vi "2D experiment wii.vi"() -> ()   [LabVIEW 2011]
uses:
  <vilib>/Platform/TimedLoop/XDataNode/timing_clust.ctl
  <vilib>/Platform/TimedLoop/XDataNode/nitl_modes.ctl
  <vilib>/Platform/TimedLoop/XDataNode/wakeup.ctl
  3D_Experiment/libs/experiments 2/Action Engines/AE Access VIs/AE - Bluetooth Initialise.vi
  3D_Experiment/libs/experiments 2/Action Engines/AE Access VIs/AE - Bluetooth Connect All.vi
  <vilib>/Utility/cursorutil.llb/Set Cursor (Cursor ID).vi
  <vilib>/Utility/inputDevices.llb/closeMouse.vi
  <vilib>/Utility/inputDevices.llb/mouseAcquire.vi
  <vilib>/Utility/file.llb/Write To Spreadsheet File (DBL).vi
  <vilib>/Utility/file.llb/Write To Spreadsheet File (I64).vi
  <vilib>/Platform/TimedLoop/XDataNode/XDataNode.xnode
  User32.dll
  <vilib>/Platform/TimedLoop/XDataNode/XDNodeRunTimeDep.lvlib
panel:
  out "initial time":u32
  out "XY Graph":cluster{"Y":dbl[], "Y":dbl[]}[](graph)
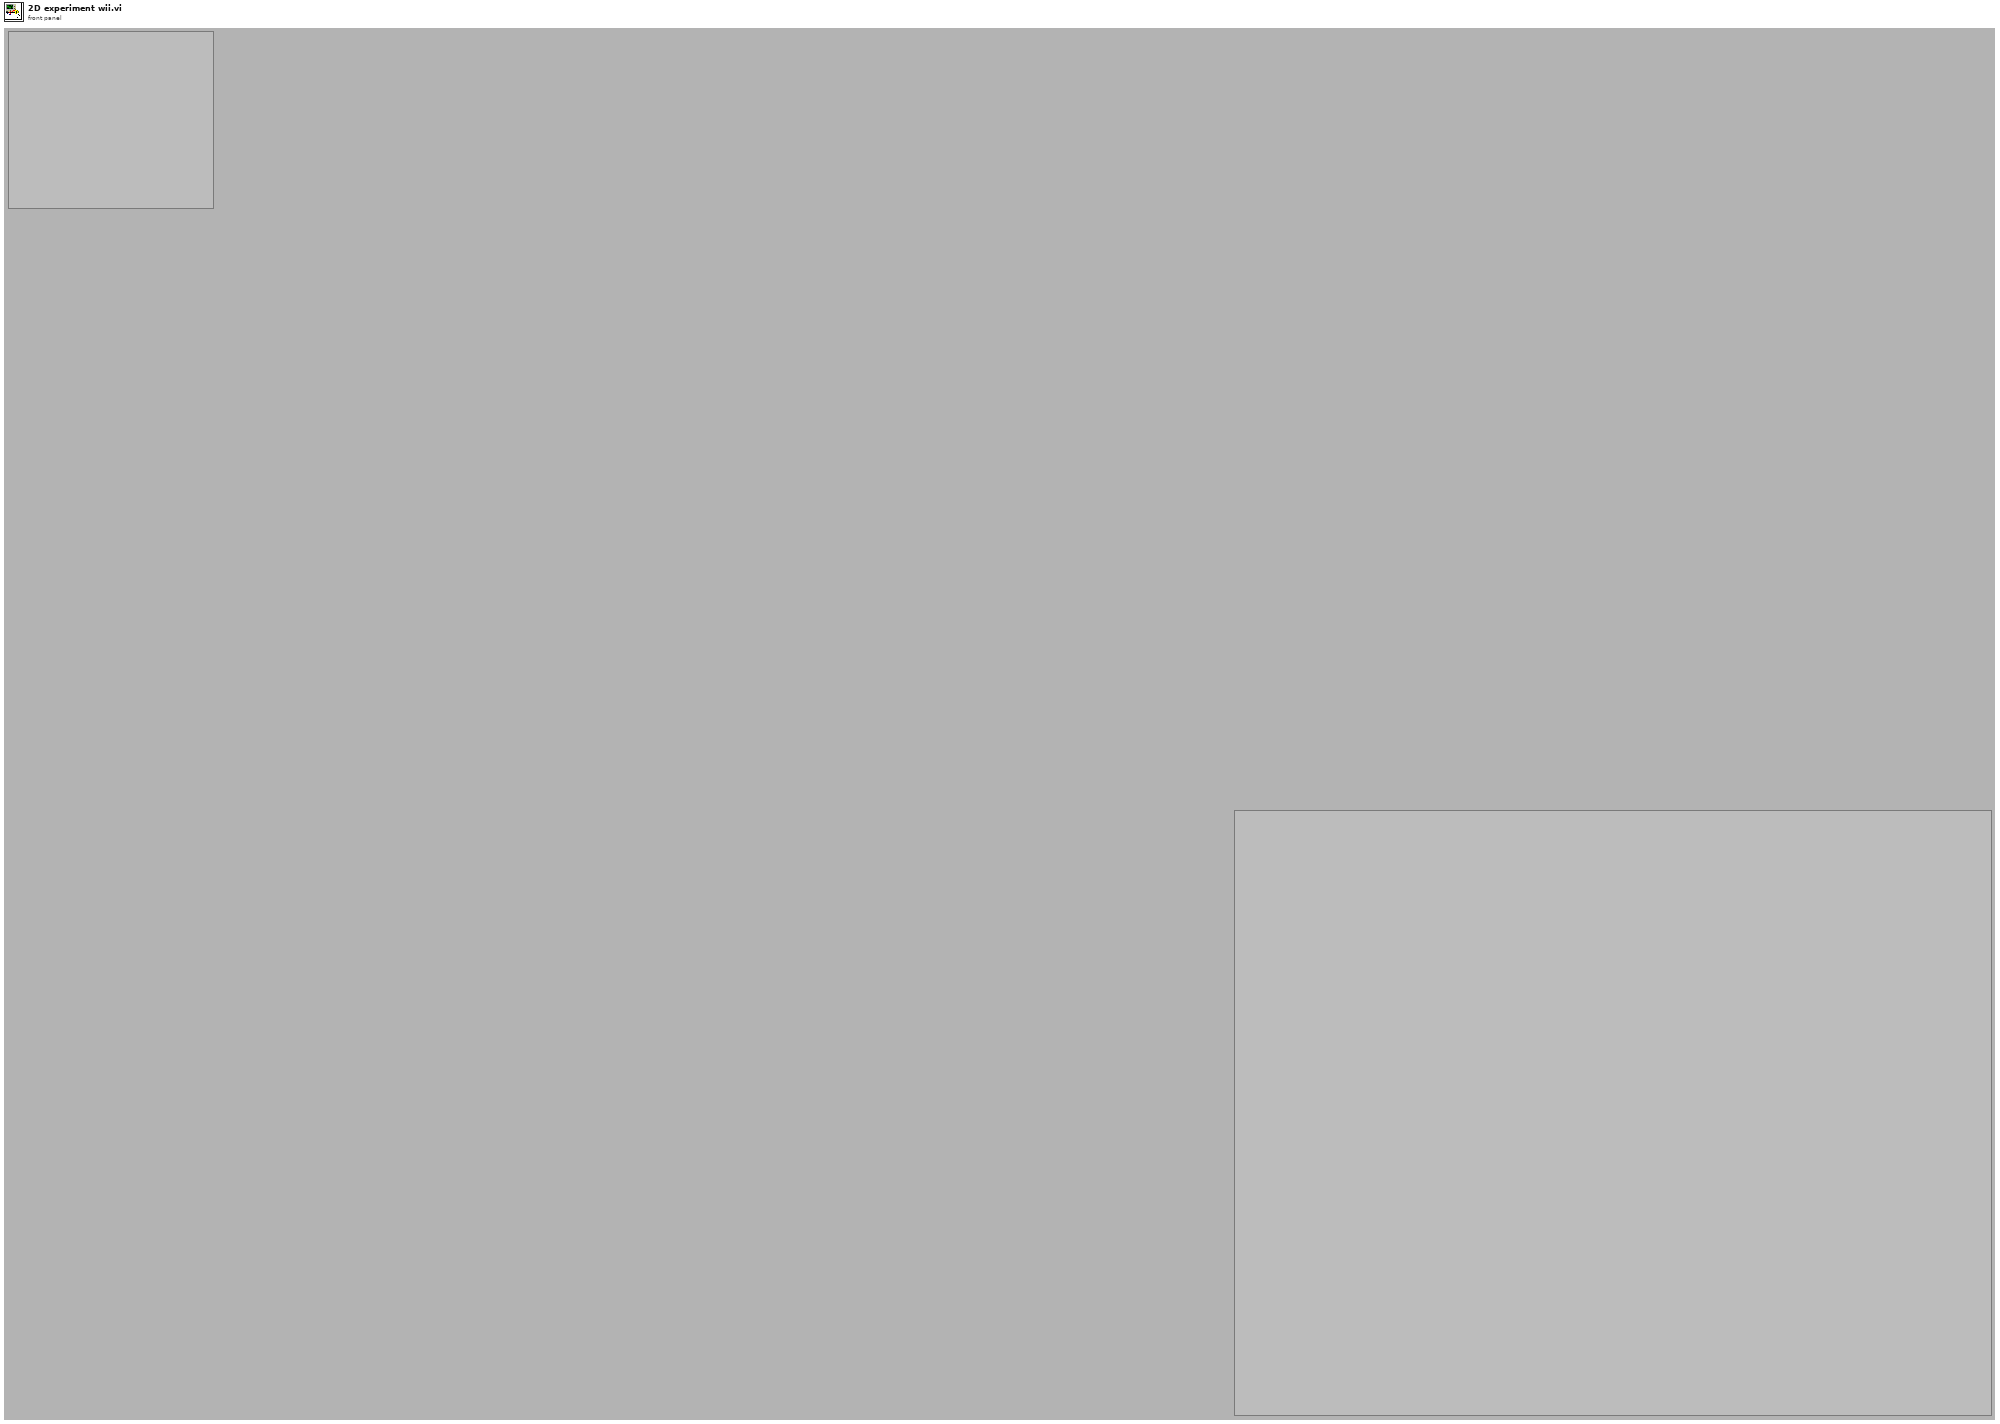
[diagram p1: front panel]
types:
  T1 = enum16{"open", "replace", "create", "open or create", "replace or create", "replace or create with confirmation"}
  T2 = typedef "XDNodeRunTimeDep.lvlib/timing_clust.ctl" = cluster{"Expected End [f-1]":u64, "Actual End [f-1]":u64, "Finished Late? [f-1]":bool, "Expected End [i-1]":u64, "Actual End [i-1]":u64, "Finished Late? [i-1]":bool, "Expected Start [i]":u64, "Actual Start [i]":u64, "Expected Start [f]":u64, "Actual Start [f]":u64, "Source Name":string, "Structure Name":string, "Period":i64, "Deadline":i64, "Offset":i64, "Start":i64, "Priority":i32, "Timeout":i32, "Mode":T3, "Wakeup Reason":T4, "Error":errorcluster, "Source Type":string, "Secondary Source Type":string, "Global End Time":u64, "Global Start Time":u64, "Frame Duration":u64, "Iteration Duration":u64, "Assigned CPU":i32, "I/O Scan Engine Mode":u32}
  T3 = typedef "XDNodeRunTimeDep.lvlib/nitl_modes.ctl" = enum32{"No Change", "Process missed periods, maintain original phase", "Discard missed periods, maintain original phase", "Process missed periods, ignore original phase", "Discard missed periods, ignore original phase"}
  T4 = typedef "XDNodeRunTimeDep.lvlib/wakeup.ctl" = enum32{"Normal", "Aborted", "Asynchronous wakeup", "Timing source error", "Timed loop error", "Timeout"}
  T5 = typedef "LVAllMonitorsDisplayTypeDef.ctl" = cluster{"Bounds":cluster{"Left":i16, "Top":i16, "Right":i16, "Bottom":i16}, "Depth":i16}[]
  T6 = cluster{"Bounds":cluster{"Left":i16, "Top":i16, "Right":i16, "Bottom":i16}, "Depth":i16}
  T7 = cluster{"Left":i16, "Top":i16, "Right":i16, "Bottom":i16}
  T8 = cluster{"Horizontal":i32, "Vertical":i32, "Scrolling":i32}
  T9 = cluster{"button 1":bool, "button 2":bool, "button 3":bool, "button 4":bool}
  T10 = cluster{"Radius":dbl, "x0":dbl, "y0":dbl, "D":dbl, bool}
  T11 = typedef "LVPoint32TypeDef.ctl" = cluster{"Horizontal":i32, "Vertical":i32}
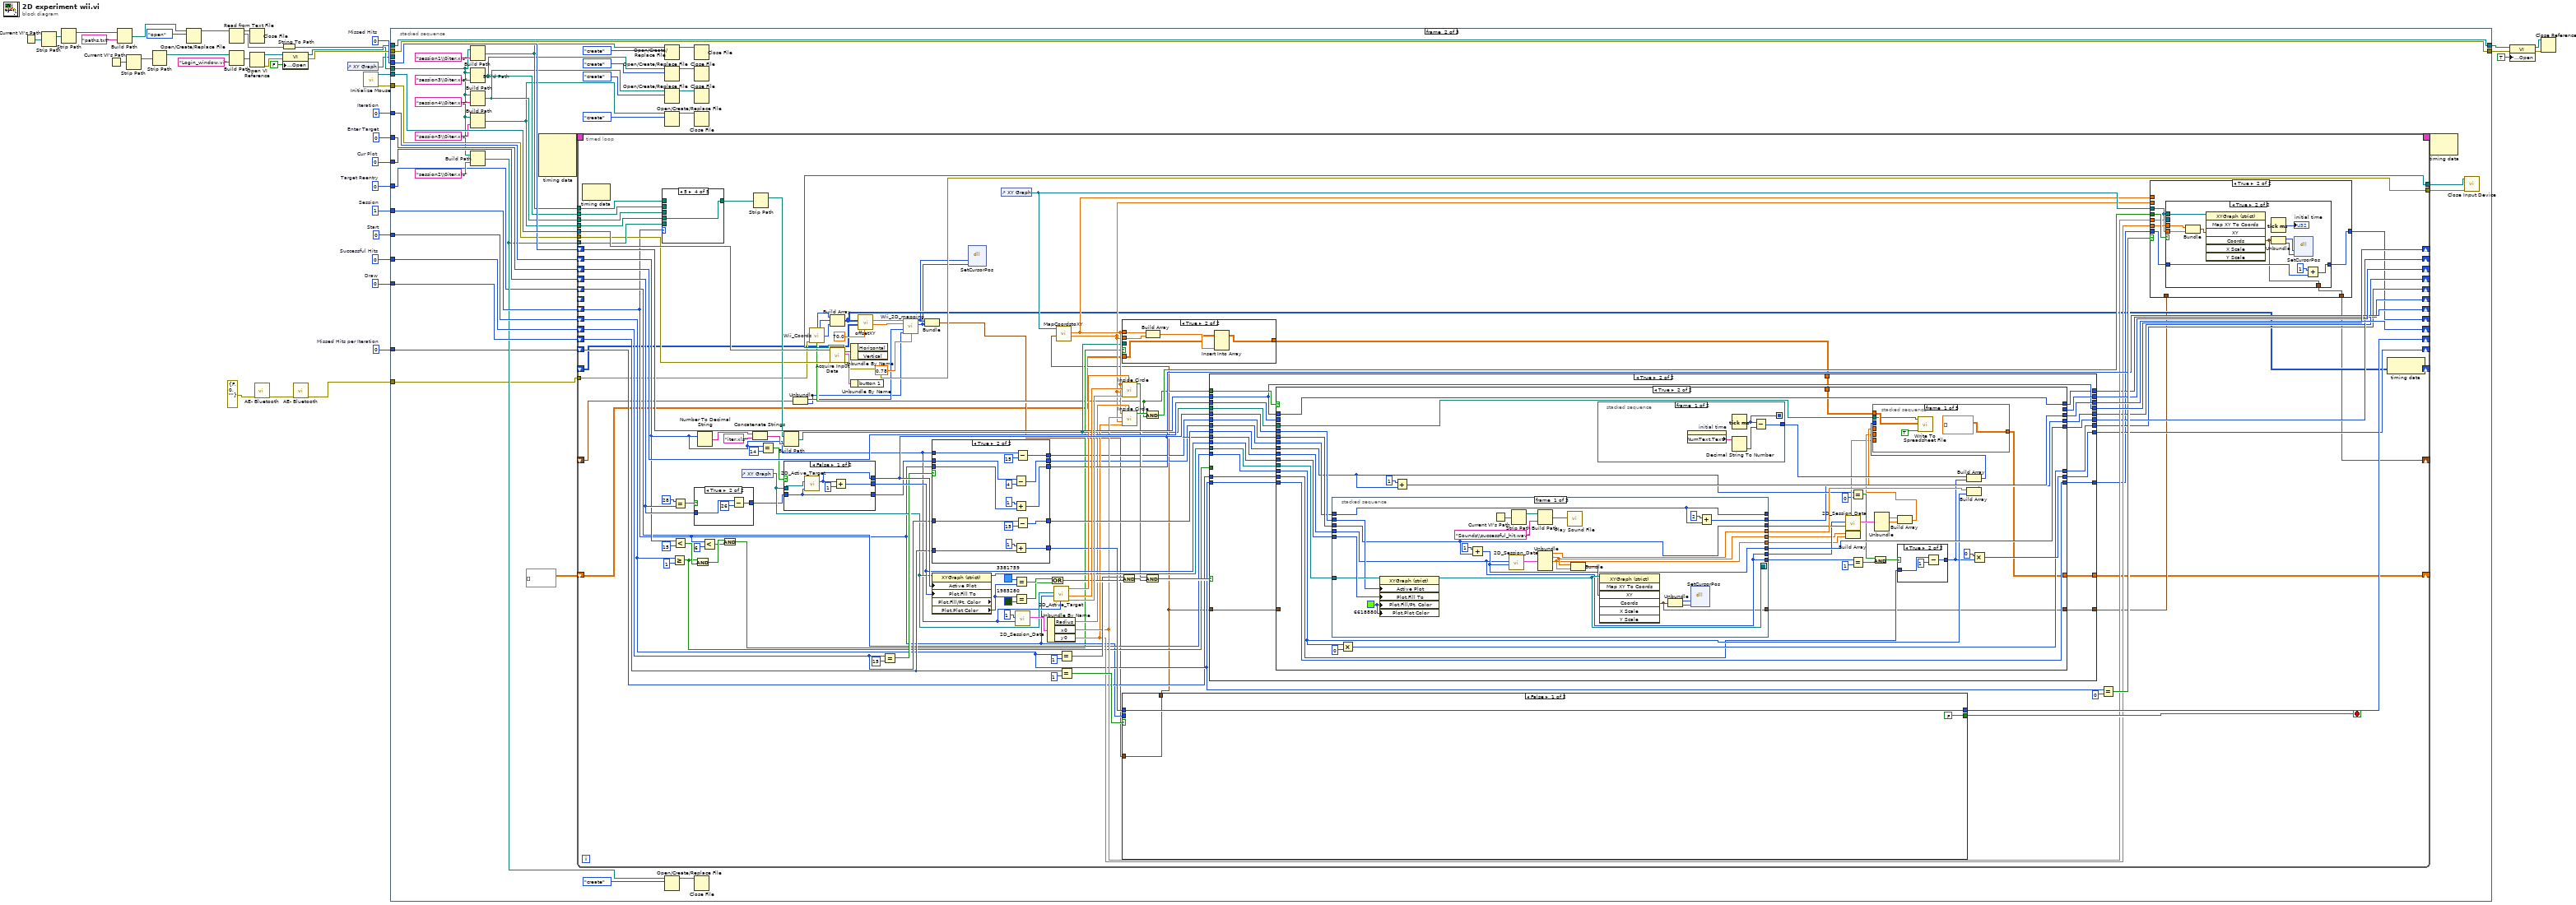
[diagram p0: block diagram]
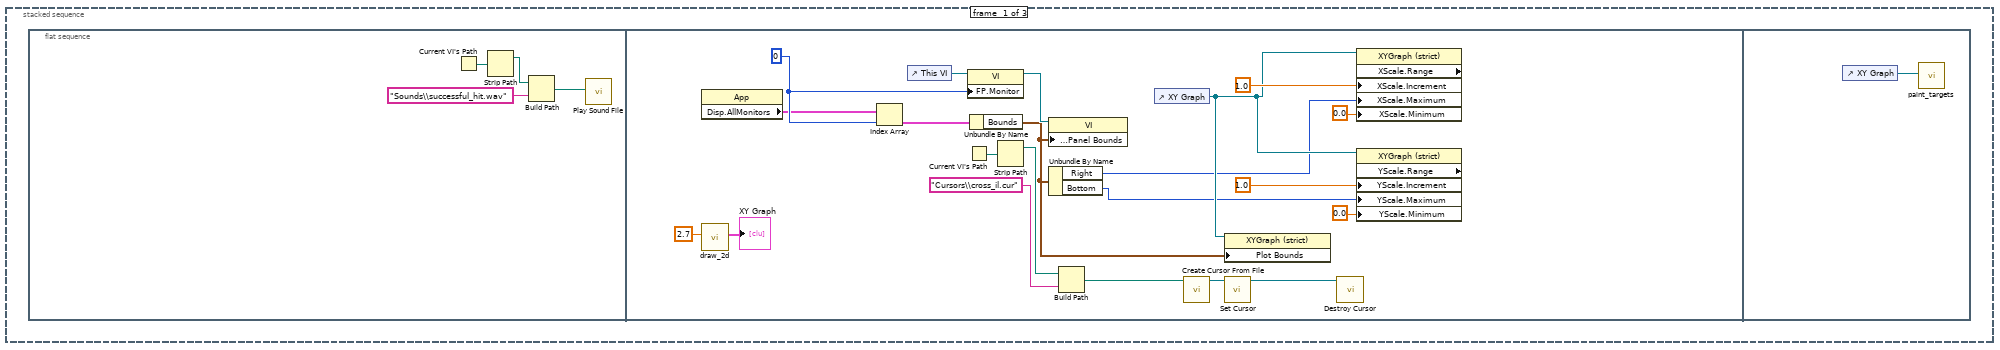
[diagram p2: hidden frame]
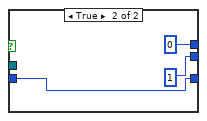
[diagram p8: hidden frame]
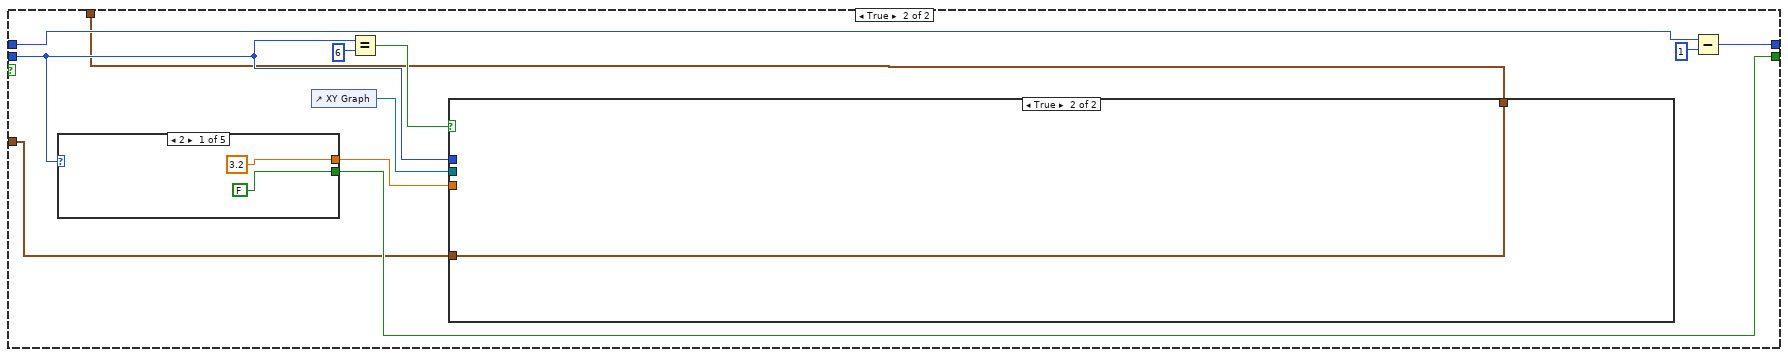
[diagram p10: hidden frame]
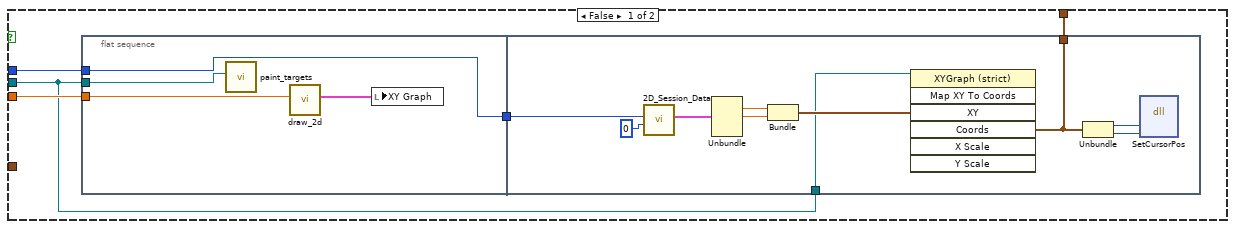
[diagram p11: hidden frame]
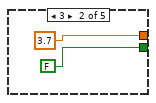
[diagram p12: hidden frame]
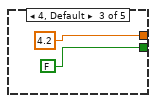
[diagram p13: hidden frame]
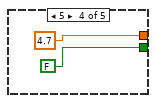
[diagram p14: hidden frame]
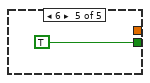
[diagram p15: hidden frame]
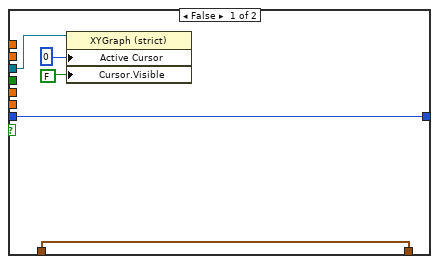
[diagram p16: hidden frame]
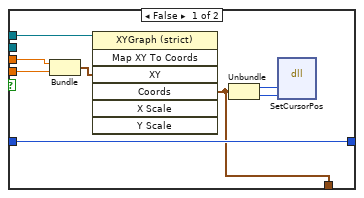
[diagram p17: hidden frame]
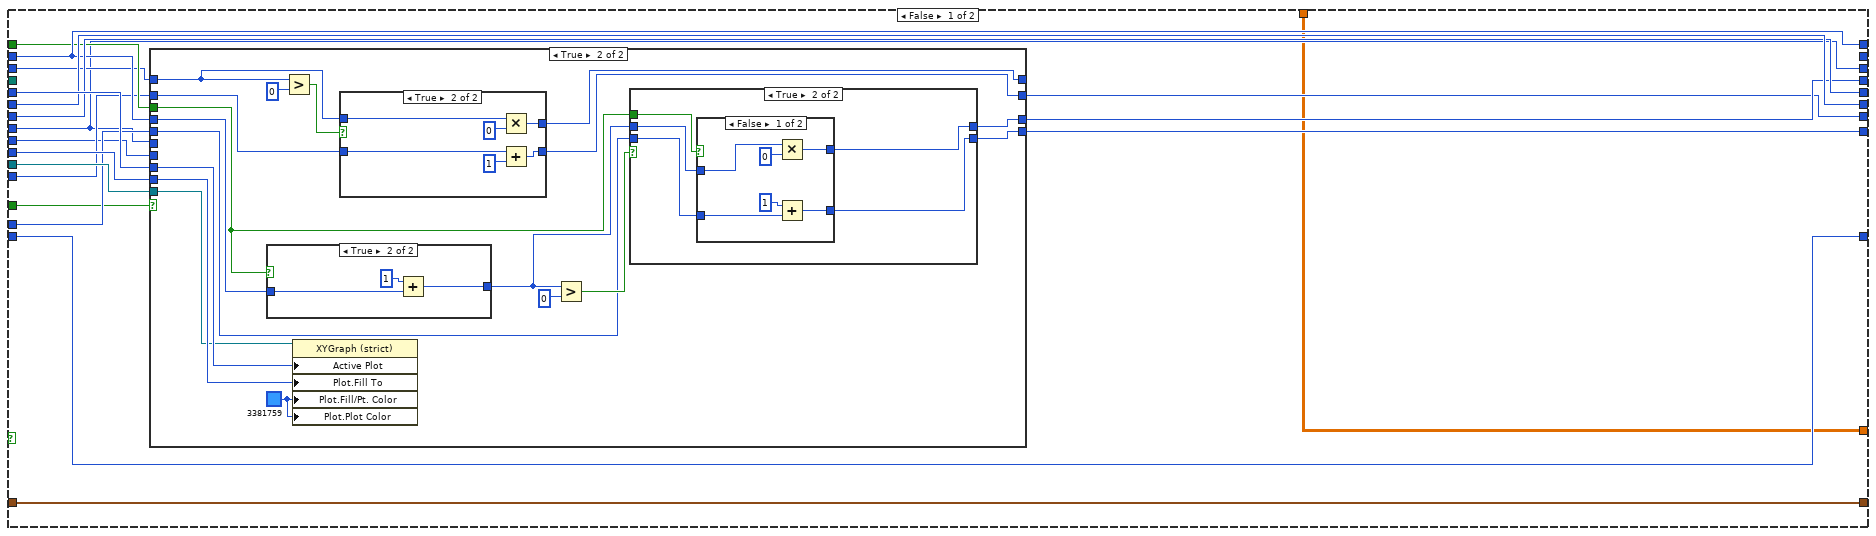
[diagram p19: hidden frame]
diagram:
  w4 = 0  # Target Reentry
  w5 = 0  # Missed Hits per Iteration
  w33 = 0  # Iteration
  w34 = 0  # Cur Plot
  w36 = 0  # Start
  w37 = 0  # Draw
  w38 = 1  # Session
  w39 = 0  # Successful Hits
  w40 = 0  # Missed Hits
  w41 = 0  # Enter Target
  n1 = Current VI's Path() -> (path=w14:path)
  n2 = Strip Path(path=w14) -> (stripped path=w9:path)  [unwired: 1 out]
  n3 = Strip Path(path=w9) -> (stripped path=w8:path)  [unwired: 1 out]
  n4 = Current VI's Path() -> (path=w29:path)
  n5 = Build Path(base path=w8, name or relative path="paths.txt") -> (appended path=w13:path)
  n6 = Strip Path(path=w29) -> (stripped path=w24:path)  [unwired: 1 out]
  n7 = Strip Path(path=w24) -> (stripped path=w23:path)  [unwired: 1 out]
  n8 = Open/Create/Replace File(file path (use dialog)=w13, operation (0:open)=T1."open") -> (refnum out=w16:refnum<file>)  [unwired: 4 in, 2 out]
  n9 = Read from Text File(file (use dialog)=w16) -> (refnum out=w17:refnum<file>, text=w15:string)  [unwired: 3 in, 2 out]
  n10 = Build Path(base path=w23, name or relative path="Login_window.vi") -> (appended path=w27:path)
  n11 = Close File(refnum=w17) -> ()  [unwired: 1 in, 2 out]
  n12 = Open VI Reference(vi path=w27) -> (vi reference=w32:refnum<vi>, error out=w31:errorcluster)  [unwired: 5 in]
  n13 = call-poly "AE- Bluetooth.vi"("error in (no error)"=errorcluster {"status"=FALSE, "code"=0, "source"=""}) -> ("error out"=w3:errorcluster)  [unwired: 10 in]
  n14 = String To Path(string=w15) -> (path=w10:path)
  n15 = property class="VI"(reference=w32, error in=w31, "Front Panel Window:Open"=FALSE) -> (reference out=w26:refnum<vi>, error out=w25:errorcluster)
  n16 = call-poly "AE- Bluetooth.vi"("error in (no error)"=w3) -> ("error out"=w2:errorcluster)  [unwired: 9 in, 1 out]
  n17 = control-ref of="XY Graph"() -> (w7:refnum<vi>)
  n18 = call <vilib>:"Initialize Mouse.vi"() -> ("error out"=w6:errorcluster, "device ID"=w35:refnum<k1>)  [unwired: 10 in]
  n19 = stacked-sequence {
    tunnel: w35 -> [_ w108 _]
    tunnel: w39 -> [_ w107 _]
    tunnel: w40 -> [_ w106 _]
    tunnel: w38 -> [_ w102 _]
    tunnel: w36 -> [_ w105 _]
    tunnel: w37 -> [_ w104 _]
    tunnel: w41 -> [_ w103 _]
    tunnel: w34 -> [_ w101 _]
    tunnel: w33 -> [_ w100 _]
    tunnel: w26 -> [_ w97 _]
    tunnel: w25 -> [_ w96 _]
    tunnel: [_ w97 _] -> w19
    tunnel: [_ w96 _] -> w18
    tunnel: w10 -> [_ w76 _]
    tunnel: w7 -> [_ _ w568]
    tunnel: w6 -> [_ w82 _]
    tunnel: w5 -> [_ w80 _]
    tunnel: w4 -> [_ w79 _]
    tunnel: w2 -> [_ w69 _]
    frame #0 {
      n20 = flat-sequence {
        frame #0 {
          n21 = Current VI's Path() -> (path=w43:path)
          n22 = Strip Path(path=w43) -> (stripped path=w44:path)  [unwired: 1 out]
          n23 = Build Path(base path=w44, name or relative path="Sounds\\successful_hit.wav") -> (appended path=w42:path)
          n24 = call <vilib>:"Play Sound File.vi"("path"=w42) -> ()  [unwired: 9 in, 2 out]
        }
        frame #1 {
          w62 = u16 0 ("Front Panel Window:Monitor")
          n25 = property class="App"() -> ("Disp.AllMonitors"=w61:T5)  [unwired: 2 in, 2 out]
          n26 = call "draw_2d.vi"("ID"=2.7) -> ("appended array"=→"XY Graph":cluster{dbl[], dbl[]}[])  [unwired: 10 in]
          n27 = Index Array(array=w61, index=w62) -> (element=w63:T6)
          n28 = control-ref of="This VI"() -> (w64:refnum<vi>)
          n29 = Current VI's Path() -> (path=w53:path)
          n30 = property class="VI"(reference=w64, "FP.Monitor"=w62) -> (reference out=w60:refnum<vi>)  [unwired: 1 in, 1 out]
          n31 = Unbundle By Name(w63) -> ("Bounds"=w59:T7)
          n32 = Strip Path(path=w53) -> (stripped path=w52:path)  [unwired: 1 out]
          n33 = property class="VI"(reference=w60, "Front Panel Window:Panel Bounds"=w59) -> ()  [unwired: 1 in, 2 out]
          n34 = Unbundle By Name(w59) -> ("Right"=w47:i16, "Bottom"=w46:i16)
          n35 = Build Path(base path=w52, name or relative path="Cursors\\cross_il.cur") -> (appended path=w50:path)
          n36 = control-ref of="XY Graph"() -> (w54:refnum<vi>)
          n37 = call <vilib>:"Create Cursor From File.vi"("cursor file"=w50) -> ("cursor ID"=w49:refnum<k1>)  [unwired: 9 in, 1 out]
          n38 = property on="Property Node" class="XYGraph (strict)"(reference=w54, "Plot Bounds"=w59) -> ()  [unwired: 1 in, 2 out]
          n39 = call-poly <vilib>:"Set Cursor.vi"("cursor ID"=w49) -> ("previous cursor ID"=w48:refnum<k1>)  [unwired: 9 in, 1 out]
          n40 = call <vilib>:"Destroy Cursor.vi"("cursor ID"=w48) -> ()  [unwired: 9 in, 1 out]
          n41 = property on="Property Node" class="XYGraph (strict)" props=["XScale", "Range", "XScale", "Increment", "XScale", "Maximum", "XScale", "Minimum"](reference=w54, "XScale.Increment"=1.0 ("X Scale.Range:Increment"), "XScale.Maximum"=w47, "XScale.Minimum"=0.0 ("X Scale.Range:Minimum")) -> ()  [unwired: 1 in, 3 out]
          n42 = property on="Property Node" class="XYGraph (strict)" props=["YScale", "Range", "YScale", "Increment", "YScale", "Maximum", "YScale", "Minimum"](reference=w54, "YScale.Increment"=1.0 ("Y Scale.Range:Increment"), "YScale.Maximum"=w46, "YScale.Minimum"=0.0 ("Y Scale.Range:Minimum")) -> ()  [unwired: 1 in, 3 out]
        }
        frame #2 {
          n43 = control-ref of="XY Graph"() -> (w67:refnum<vi>)
          n44 = call "paint_targets.vi"("XYGraph Refnum"=w67) -> ()  [unwired: 11 in]
        }
      }
    }
    frame #1 {
      n45 = Build Path(base path=w76, name or relative path="session1\\0iter.xls") -> (appended path=w90:path)
      n46 = Build Path(base path=w76, name or relative path="session3\\0iter.xls") -> (appended path=w84:path)
      n47 = Build Path(base path=w76, name or relative path="session4\\0iter.xls") -> (appended path=w73:path)
      n48 = Build Path(base path=w76, name or relative path="session5\\0iter.xls") -> (appended path=w70:path)
      n49 = Build Path(base path=w76, name or relative path="session2\\0iter.xls") -> (appended path=w87:path)
      n50 = node-c288() -> (w99:T2)  [unwired: 4 in]
      n51 = timed-loop {
        tunnel: w108 -> [w213]
        tunnel: [w212] -> w83
        shift-right: [w211] -> _
        shift-left: w107 -> [w198]
        shift-right: [w209] -> _
        shift-left: w106 -> [w210]
        shift-right: [w190] -> _
        shift-left: w102 -> [w137]
        shift-right: [w139] -> _
        shift-left: w105 -> [w158]
        shift-right: [w195] -> _
        shift-left: w104 -> [w196]
        shift-right: [w191] -> _
        shift-left: w103 -> [w192]
        shift-right: [w175] -> _
        shift-left: w100 -> [w149]
        shift-right: [w174] -> _
        shift-left: w101 -> [w171]
        timing: w99 -> [_]
        timing-out: [_] -> w98
        tunnel: w90 -> [w164]
        tunnel: w87 -> [w163]
        tunnel: w84 -> [w162]
        shift-right: [w151] -> _
        shift-left: _ -> [_]
        tunnel: w82 -> [w147]
        tunnel: [w146] -> w81
        shift-right: [w144] -> _
        shift-left: w80 -> [w145]
        shift-right: [w141] -> _
        shift-left: w79 -> [w143]
        tunnel: w73 -> [w133]
        tunnel: w70 -> [w132]
        tunnel: w69 -> [w123]
        shift-right: [w122] -> _
        shift-left: _ -> [w121]
        shift-right: [w117] -> _
        shift-left: _ -> [w116]
        shift-right: [w109] -> _
        shift-left: dbl[][] [] -> [w111]
        stop <- w184 stop-if-true
        n52 = node-c288() -> ()  [unwired: 1 in, 1 out]
        n53 = case shown="5" w137 {
          tunnel: w164 -> [_ _ _ _ w234]
          tunnel: [w230 w231 w232 w233 w234] -> w157
          tunnel: w163 -> [w230 _ _ _ _]
          tunnel: w162 -> [_ w231 _ _ _]
          tunnel: w133 -> [_ _ w232 _ _]
          tunnel: w132 -> [_ _ _ w233 _]
          frame 2 {
          }
          frame 3 {
          }
          frame 4 {
          }
          frame 5 {
          }
          frame 1, Default {
          }
        }
        n54 = Greater Or Equal?(x=w158, y=1) -> (x >= y?=w142:bool)
        n55 = Equal?(x=28, y=w171) -> (x = y?=w172:bool)
        n56 = Less?(x=w149, y=15) -> (x < y?=w148:bool)
        n57 = case shown="True" w172 {
          tunnel: w171 -> [w245 w248]
          tunnel: [w245 w246] -> w170
          frame False {
          }
          frame True {
            n58 = Subtract(x=w248, y=26) -> (x-y=w246:i32)
          }
        }
        n59 = And(x=w142, y=w148) -> (x .and. y?=w138:bool)
        n60 = Number To Decimal String(number=w149) -> (decimal integer string=w153:string)  [unwired: 1 in]
        n61 = Less?(x=w137, y=6) -> (x < y?=w135:bool)
        n62 = And(x=w138, y=w135) -> (x .and. y?=w134:bool)
        n63 = control-ref of="XY Graph"() -> (w178:refnum<vi>)
        n64 = Concatenate Strings(w153, "iter.xls" ("name or relative path")) -> (w155:string)
        n65 = Strip Path(path=w157) -> (stripped path=w154:path)  [unwired: 1 out]
        n66 = Equal?(x=w149, y=14) -> (x = y?=w168:bool)
        n67 = Build Path(base path=w154, name or relative path=w155) -> (appended path=w152:path)
        n68 = case shown="False" w168 {
          tunnel: [w240 u32 0 ("Active Plot")] -> w218
          tunnel: [w239 u32 1] -> w217
          tunnel: w178 -> [w238 _]
          tunnel: w170 -> [w237 w242]
          tunnel: [w237 w242] -> w167
          frame False {
            n69 = call "2D_Active_Target.vi"("Active Plot"=w237, "XYGraph Refnum"=w238) -> ("Active Plot"=w240:u32)  [unwired: 6 in, 3 out]
            n70 = Add(x=w240, y=u32 1) -> (x+y=w239:u32)
          }
          frame True {
          }
        }
        n71 = Unbundle(w116) -> ("Horizontal"=w115:i32, "Vertical"=w114:i32)
        n72 = call "Wii_Coords.vi"("error in (no error)"=w123) -> ("Raw X Values"=w126:i32[], "Raw Y Values"=w125:i32[], "Sizes"=w131:i32[], "B"=w124:bool)  [unwired: 7 in, 4 out]
        n73 = Build Array(w126, w125, w131) -> (w122:i32[][])
        n74 = call-poly <vilib>:"Acquire Input Data.vi"("device ID"=w213, "error in (no error)"=w147) -> ("device ID"=w212:refnum<k1>, "axis info"=w177:T8, "button info"=w214:T9, "error out"=w146:errorcluster)  [unwired: 1 in, 13 out]
        n75 = Unbundle By Name(w177) -> ()  [unwired: 2 out]
        n76 = Unbundle By Name(w214) -> ()  [unwired: 1 out]
        n77 = call "offsetXY.vi"("Thres"=70.0, "Previous"=w121, "Current"=w122) -> ("OffsetY"=w129:dbl, "OffsetX"=w128:dbl)  [unwired: 7 in]
        n78 = Equal?(x=w198, y=15) -> (x = y?=w207:bool)
        n79 = call "Wii_2D_mapping.vi"("Wii_X_off"=w128, "Wii_Y_off"=w129, "previous_X"=w115, "previous_Y"=w114, "X_Y_speed"=0.78) -> ("X"=w120:i32, "Y"=w119:i32)  [unwired: 9 in]
        n80 = Bundle("X"=w120, "Y"=w119) -> (w113:cluster{"X":i32, "Y":i32})  [unwired: 1 in]
        n81 = case shown="True" w207 {
          tunnel: w198 -> [w327 w342]
          tunnel: [w327 w341] -> w206
          tunnel: w137 -> [w326 w340]
          tunnel: [w326 w338] -> w190
          tunnel: w196 -> [w325 w337]
          tunnel: [w325 w335] -> w194
          tunnel: w167 -> [w324 w334]
          tunnel: [w324 w332] -> w166
          tunnel: w149 -> [w323 w331]
          tunnel: [w323 w329] -> w165
          frame False {
          }
          frame True {
            n82 = Subtract(x=w334, y=4) -> (x-y=w332:i32)
            n83 = Add(x=1, y=w340) -> (x+y=w338:i32)
            n84 = Add(x=1, y=w337) -> (x+y=w335:i32)
            n85 = Subtract(x=w331, y=15) -> (x-y=w329:i32)
            n86 = Subtract(x=w342, y=15) -> (x-y=w341:i32)
          }
        }
        n87 = property on="Property Node" class="XYGraph (strict)" props=["Active Plot", "Plot", "Fill To", "Plot", "Fill/Pt. Color", "Plot", "Plot Color"](reference=w178, "Active Plot"=w218, "Plot.Fill To"=w217) -> (reference out=w199:refnum<vi>, "Plot.Plot Color"=w200:u32)  [unwired: 1 in, 2 out]
        n88 = dll-call lib="User32.dll" fn="SetCursorPos"(w120, w119) -> ()  [unwired: 6 in, 2 out]
        n89 = control-ref of="XY Graph"() -> (w176:refnum<vi>)
        n90 = Equal?(x=u32 3381759, y=w200) -> (x = y?=w220:bool)
        n91 = Equal?(x=w200, y=u32 1985280) -> (x = y?=w219:bool)
        n92 = call "2D_Session_Data.vi"("Iteration"=w149, "Session"=1) -> ("output cluster"=w183:T10)  [unwired: 9 in]
        n93 = Unbundle By Name(w183) -> ("Radius"=w182:dbl, "x0"=w181:dbl, "y0"=w180:dbl)
        n94 = Or(x=w220, y=w219) -> (x .or. y?=w188:bool)
        n95 = call "2D_Active_Target.vi"("Iteration"=w149, "Session"=w137, "XYGraph Refnum"=w178) -> ("y0"=w215:dbl, "x0"=w216:dbl, "Radius"=w205:dbl)  [unwired: 5 in, 1 out]
        n96 = Equal?(x=w158, y=1) -> (x = y?=w186:bool)
        n97 = Equal?(x=w196, y=1) -> (x = y?=w193:bool)
        n98 = And(x=w186, y=w188) -> (x .and. y?=w185:bool)
        n99 = case shown="False" w193 {
          tunnel: w137 -> [_ w254]
          tunnel: [w250 w261] -> w195
          tunnel: w194 -> [w250 w260]
          tunnel: [FALSE ("Valid") w258] -> w184
          tunnel: w113 -> [w249 w252]
          tunnel: [w249 w253] -> w112
          frame False {
          }
          frame True {
            n100 = case shown="2" w254 {
              tunnel: [3.2 ("ID") 3.7 ("ID") 4.2 ("ID") 4.7 ("ID") _] -> w259
              tunnel: [FALSE FALSE FALSE FALSE TRUE] -> w258
              frame 2 {
              }
              frame 3 {
              }
              frame 4, Default {
              }
              frame 5 {
              }
              frame 6 {
              }
            }
            n101 = control-ref of="XY Graph"() -> (w255:refnum<vi>)
            n102 = Equal?(x=w254, y=6) -> (x = y?=w256:bool)
            n103 = case shown="True" w256 {
              tunnel: w259 -> [w267 _]
              tunnel: w255 -> [w264 _]
              tunnel: w254 -> [w265 _]
              tunnel: [w263 w282] -> w253
              tunnel: w252 -> [_ w282]
              frame False {
                n104 = flat-sequence {
                  tunnel: w267 -> [w270]
                  tunnel: w264 -> [w269]
                  tunnel: [w268] -> w266
                  tunnel: w265 -> [w268]
                  tunnel: w266 -> [w275]
                  tunnel: w264 -> [w273]
                  tunnel: [w272] -> w263
                  frame #0 {
                    n105 = call "paint_targets.vi"("XYGraph Refnum"=w269) -> ()  [unwired: 11 in]
                    n106 = call "draw_2d.vi"("ID"=w270) -> ("appended array"=w271:cluster{dbl[], dbl[]}[])  [unwired: 10 in]
                    n107 = local write "XY Graph"(w271) -> ()
                  }
                  frame #1 {
                    n108 = call "2D_Session_Data.vi"("Iteration"=0, "Session"=w275) -> ("output cluster"=w279:T10)  [unwired: 9 in]
                    n109 = Unbundle(w279) -> ("x0"=w278:dbl, "y0"=w276:dbl)  [unwired: 3 out]
                    n110 = Bundle("x0"=w278, "y0"=w276) -> (w277:cluster{"x0":dbl, "y0":dbl})  [unwired: 1 in]
                    n111 = invoke on="Invoke Node" class="XYGraph (strict)" method="Map XY To Coords"(reference=w273, "XY"=w277) -> ("Coords"=w272:T11)  [unwired: 5 in, 6 out]
                    n112 = Unbundle(w272) -> ("Horizontal"=w281:i32, "Vertical"=w280:i32)
                    n113 = dll-call lib="User32.dll" fn="SetCursorPos"(w281, w280) -> ()  [unwired: 6 in, 2 out]
                  }
                }
              }
              frame True {
              }
            }
            n114 = Subtract(x=w260, y=1) -> (x-y=w261:i32)
          }
        }
        n115 = call "MapCoordstoXY.vi"("Coordinates"=w112, "XYGraph Refnum"=w176) -> ("Y(graph)"=w160:dbl, "X (graph)"=w161:dbl)  [unwired: 7 in]
        n116 = case shown="True" w134 {
          tunnel: w161 -> [_ w229]
          tunnel: w160 -> [_ w228]
          tunnel: w152 -> [_ _]
          tunnel: w111 -> [w224 w226]
          tunnel: [w224 w225] -> w110
          frame False {
          }
          frame True {
            n117 = Build Array(w229, w228) -> (w227:dbl[])
            n118 = Insert Into Array(array=w226, new element=w227) -> (w225:dbl[][])  [unwired: 2 in]
          }
        }
        n119 = call "Inside Circle.vi"("Radius"=w205, "y0"=w215, "y"=w160, "x0"=w216, "x"=w161) -> ("Inside Circle"=w187:bool)  [unwired: 6 in]
        n120 = call "Inside Circle.vi"("Radius"=w182, "y0"=w180, "y"=w160, "x0"=w181, "x"=w161) -> ("Inside Circle"=w202:bool)  [unwired: 6 in]
        n121 = And(x=w202, y=w124) -> (x .and. y?=w201:bool)
        n122 = And(x=w187, y=w185) -> (x .and. y?=w222:bool)
        n123 = case shown="True" w222 {
          tunnel: w124 -> [w353 w436]
          tunnel: w218 -> [w361 w433]
          tunnel: w217 -> [w360 w432]
          tunnel: w206 -> [w345 w435]
          tunnel: [w345 w434] -> w211
          tunnel: w210 -> [w355 w420]
          tunnel: [w351 w420] -> w209
          tunnel: w158 -> [w359 w431]
          tunnel: [w359 w430] -> w140
          tunnel: w199 -> [w358 w429]
          tunnel: w192 -> [w350 w428]
          tunnel: [_ w427] -> w191
          tunnel: w190 -> [w346 w426]
          tunnel: w165 -> [w357 w425]
          tunnel: [w357 w424] -> w175
          tunnel: w166 -> [w356 w423]
          tunnel: [w356 w422] -> w174
          tunnel: w152 -> [_ w421]
          tunnel: [w355 w419] -> w151
          tunnel: w145 -> [w354 w418]
          tunnel: [w352 w417] -> w144
          tunnel: w143 -> [w348 w416]
          tunnel: w142 -> [w349 _]
          tunnel: [w347 w415] -> w141
          tunnel: [w344 w414] -> w118
          tunnel: w112 -> [w344 w413]
          tunnel: w110 -> [w343 w412]
          tunnel: [w343 w411] -> w109
          frame False {
            n124 = case shown="True" w349 {
              tunnel: w361 -> [_ w382]
              tunnel: w360 -> [_ w381]
              tunnel: w358 -> [_ w380]
              tunnel: w355 -> [w365 w379]
              tunnel: w354 -> [w364 w375]
              tunnel: w353 -> [_ w366]
              tunnel: [w364 w374] -> w352
              tunnel: [w365 w373] -> w351
              tunnel: w350 -> [w362 w370]
              tunnel: w348 -> [w363 w369]
              tunnel: [w363 w368] -> w347
              tunnel: [w362 w367] -> _
              tunnel: w346 -> [_ _]
              tunnel: w345 -> [_ _]
              frame False {
              }
              frame True {
                w383 = u32 3381759
                n125 = case shown="True" w366 {
                  tunnel: w379 -> [w407 w410]
                  tunnel: [w407 w408] -> w376
                  frame False {
                  }
                  frame True {
                    n126 = Add(x=1, y=w410) -> (x+y=w408:i32)
                  }
                }
                n127 = Greater?(x=w370, y=0) -> (0:w371:bool)
                n128 = property on="Property Node" class="XYGraph (strict)"(reference=w380, "Active Plot"=w382, "Plot.Fill To"=w381, "Plot.Fill/Pt. Color"=w383, "Plot.Plot Color"=w383) -> ()  [unwired: 1 in, 2 out]
                n129 = case shown="True" w371 {
                  tunnel: w370 -> [w384 w391]
                  tunnel: w369 -> [w385 w388]
                  tunnel: [w385 w387] -> w368
                  tunnel: [w384 w386] -> w367
                  frame False {
                  }
                  frame True {
                    n130 = Multiply(x=w391, y=0) -> (x*y=w386:i32)
                    n131 = Add(x=w388, y=1) -> (x+y=w387:i32)
                  }
                }
                n132 = Greater?(x=w376, y=0) -> (0:w377:bool)
                n133 = case shown="True" w377 {
                  tunnel: [w392 w398] -> w374
                  tunnel: [w393 w397] -> w373
                  tunnel: w376 -> [w393 w396]
                  tunnel: w375 -> [w392 w395]
                  tunnel: w366 -> [_ w394]
                  frame False {
                  }
                  frame True {
                    n134 = case shown="False" w394 {
                      tunnel: [w403 w405] -> w398
                      tunnel: [w401 w406] -> w397
                      tunnel: w396 -> [w400 w406]
                      tunnel: w395 -> [w399 w405]
                      frame False {
                        n135 = Multiply(x=w400, y=0) -> (x*y=w401:i32)
                        n136 = Add(x=1, y=w399) -> (x+y=w403:i32)
                      }
                      frame True {
                      }
                    }
                  }
                }
              }
            }
          }
          frame True {
            n137 = case shown="True" w436 {
              tunnel: w435 -> [w451 w465]
              tunnel: [w451 w490] -> w434
              tunnel: w433 -> [w450 w494]
              tunnel: w432 -> [w449 w493]
              tunnel: w431 -> [w448 w492]
              tunnel: [w448 w492] -> w430
              tunnel: w429 -> [w447 w491]
              tunnel: w428 -> [w446 _]
              tunnel: [w444 _] -> w427
              tunnel: w426 -> [_ w489]
              tunnel: w425 -> [w443 w488]
              tunnel: [w443 w487] -> w424
              tunnel: w423 -> [w442 w486]
              tunnel: [w442 w456] -> w422
              tunnel: w421 -> [_ w483]
              tunnel: w420 -> [w441 w482]
              tunnel: [w441 w482] -> w419
              tunnel: w418 -> [w440 w458]
              tunnel: [w440 w481] -> w417
              tunnel: w416 -> [w439 w478]
              tunnel: [w439 w476] -> w415
              tunnel: [w438 w455] -> w414
              tunnel: w413 -> [w438 _]
              tunnel: w412 -> [w437 w454]
              tunnel: [w437 w453] -> w411
              frame False {
                w452 = u32 1985280
                n138 = property on="Property Node" class="XYGraph (strict)"(reference=w447, "Active Plot"=w450, "Plot.Fill To"=w449, "Plot.Fill/Pt. Color"=w452, "Plot.Plot Color"=w452) -> ()  [unwired: 1 in, 2 out]
                n139 = Add(x=w446, y=1) -> (x+y=w444:i32)
              }
              frame True {
                n140 = stacked-sequence {
                  seq-local: [w542 _ _] -> [_ w551 w562]
                  tunnel: w494 -> [w541 w550 w564]
                  tunnel: w493 -> [w544 _ w563]
                  tunnel: w491 -> [w543 _ _]
                  tunnel: w489 -> [w523 _ _]
                  tunnel: w488 -> [w526 w549 _]
                  tunnel: [w528 _ _] -> w487
                  tunnel: [w535 _ _] -> _
                  tunnel: w486 -> [w535 _ _]
                  tunnel: [w533 _ _] -> w456
                  tunnel: [w527 _ _] -> w479
                  tunnel: [w526 _ _] -> w474
                  tunnel: [w523 _ _] -> w473
                  tunnel: [w525 _ _] -> w469
                  tunnel: [w524 _ _] -> w468
                  tunnel: [w523 _ _] -> w463
                  tunnel: [w522 _ _] -> w455
                  frame #0 {
                    w545 = u32 6618880
                    n141 = property on="Property Node" class="XYGraph (strict)"(reference=w543, "Active Plot"=w541, "Plot.Fill To"=w544, "Plot.Fill/Pt. Color"=w545, "Plot.Plot Color"=w545) -> (reference out=w542:refnum<vi>)  [unwired: 1 in, 1 out]
                    n142 = Add(x=1, y=w526) -> (x+y=w528:i32)
                    n143 = Current VI's Path() -> (path=w538:path)
                    n144 = call "2D_Session_Data.vi"("Iteration"=w528, "Session"=w523) -> ("output cluster"=w530:T10)  [unwired: 9 in]
                    n145 = Strip Path(path=w538) -> (stripped path=w537:path)  [unwired: 1 out]
                    n146 = Build Path(base path=w537, name or relative path="Sounds\\successful_hit.wav") -> (appended path=w539:path)
                    n147 = Unbundle(w530) -> ("Radius"=w527:dbl, "x0"=w525:dbl, "y0"=w524:dbl)  [unwired: 2 out]
                    n148 = call <vilib>:"Play Sound File.vi"("path"=w539) -> ()  [unwired: 9 in, 2 out]
                    n149 = Bundle("x0"=w525, "y0"=w524) -> (w529:cluster{"x0":dbl, "y0":dbl})  [unwired: 1 in]
                    n150 = invoke on="Invoke Node" class="XYGraph (strict)" method="Map XY To Coords"(reference=w542, "XY"=w529) -> ("Coords"=w522:T11)  [unwired: 5 in, 6 out]
                    n151 = Unbundle(w522) -> ("Horizontal"=w532:i32, "Vertical"=w531:i32)
                    n152 = dll-call lib="User32.dll" fn="SetCursorPos"(w532, w531) -> ()  [unwired: 6 in, 2 out]
                    n153 = Add(x=2, y=w535) -> (x+y=w533:i32)
                  }
                  frame #1 {
                    w553 = u32 3381759
                    n154 = Equal?(x=15, y=w549) -> (x = y?=w547:bool)
                    n155 = case shown="True" w547 {
                      tunnel: [w555 w559] -> w552
                      tunnel: w550 -> [w554 w561]
                      tunnel: [w554 w557] -> w546
                      frame False {
                        n156 = Add(x=w554, y=u32 1) -> (x+y=w555:u32)
                      }
                      frame True {
                        n157 = Subtract(x=w561, y=u32 2) -> (x-y=w557:u32)
                        n158 = Add(x=w557, y=1 ("x")) -> (x+y=w559:u32)
                      }
                    }
                    n159 = property on="Property Node" class="XYGraph (strict)"(reference=w551, "Active Plot"=w546, "Plot.Fill To"=w552, "Plot.Fill/Pt. Color"=w553, "Plot.Plot Color"=w553) -> ()  [unwired: 1 in, 2 out]
                  }
                  frame #2 {
                    w565 = u32 3223857
                    n160 = property on="Property Node" class="XYGraph (strict)"(reference=w562, "Active Plot"=w564, "Plot.Fill To"=w563, "Plot.Fill/Pt. Color"=w565, "Plot.Plot Color"=w565) -> ()  [unwired: 1 in, 2 out]
                  }
                }
                n161 = Multiply(x=w478, y=0) -> (x*y=w476:i32)
                n162 = Add(x=1, y=w465) -> (x+y=w490:i32)
                n163 = stacked-sequence {
                  seq-local: [w516 _] -> [_ w520]
                  tunnel: [w517 _] -> w484
                  frame #0 {
                    n164 = property on="initial time" class="DigNum (strict)"() -> ("NumText.Text"=w519:string)  [unwired: 2 in, 2 out]
                    n165 = Tick Count (ms)() -> (millisecond timer value=w516:u32)
                    n166 = Decimal String To Number(string=w519) -> (number=w518:i32)  [unwired: 2 in, 1 out]
                    n167 = Subtract(x=w516, y=w518) -> (x-y=w517:u32)
                  }
                  frame #1 {
                    n168 = Number To Decimal String(number=w520) -> (decimal integer string=w521:string)  [unwired: 1 in]
                    n169 = property on="initial time" class="DigNum (strict)"("NumText.Text"=w521) -> ()  [unwired: 2 in, 2 out]
                  }
                }
                n170 = Build Array(w469, w468) -> (w466:dbl[])
                n171 = call "2D_Session_Data.vi"("Iteration"=w474, "Session"=w473) -> ("output cluster"=w472:T10)  [unwired: 9 in]
                n172 = Equal?(x=w465, y=0) -> (x = y?=w461:bool)
                n173 = Equal?(x=w463, y=1) -> (x = y?=w460:bool)
                n174 = And(x=w461, y=w460) -> (x .and. y?=w459:bool)
                n175 = Unbundle(w472) -> ("x0"=w471:dbl, "y0"=w470:dbl)  [unwired: 3 out]
                n176 = Build Array(w471, w470) -> (w467:dbl[])
                n177 = case shown="True" w459 {
                  tunnel: w458 -> [w496 w498]
                  tunnel: [w496 w497] -> w457
                  frame False {
                  }
                  frame True {
                    n178 = Subtract(x=w498, y=1) -> (x-y=w497:i32)
                  }
                }
                n179 = Build Array(w484, w457) -> (w485:u32[])
                n180 = Build Array(w479, w478) -> (w475:dbl[])
                n181 = stacked-sequence {
                  tunnel: w485 -> [_ w506 _ _ _]
                  tunnel: w483 -> [w501 w504 w507 w512 w514]
                  tunnel: w475 -> [_ _ w509 _ _]
                  tunnel: w467 -> [_ _ _ w511 _]
                  tunnel: w466 -> [_ _ _ _ w515]
                  tunnel: w454 -> [w502 _ _ _ _]
                  tunnel: [dbl[][] [] _ _ _ _] -> w453
                  frame #0 {
                    n182 = call-poly <vilib>:"Write To Spreadsheet File.vi"("append to file? (new file:F)"=TRUE, "2D data"=w502, "file path (dialog if empty)"=w501) -> ()  [unwired: 5 in, 1 out]
                  }
                  frame #1 {
                    n183 = call-poly <vilib>:"Write To Spreadsheet File.vi"("append to file? (new file:F)"=TRUE, "1D data"=w506, "file path (dialog if empty)"=w504) -> ()  [unwired: 5 in, 1 out]
                  }
                  frame #2 {
                    n184 = call-poly <vilib>:"Write To Spreadsheet File.vi"("append to file? (new file:F)"=TRUE, "1D data"=w509, "file path (dialog if empty)"=w507) -> ()  [unwired: 5 in, 1 out]
                  }
                  frame #3 {
                    n185 = call-poly <vilib>:"Write To Spreadsheet File.vi"("append to file? (new file:F)"=TRUE, "1D data"=w511, "file path (dialog if empty)"=w512) -> ()  [unwired: 5 in, 1 out]
                  }
                  frame #4 {
                    n186 = call-poly <vilib>:"Write To Spreadsheet File.vi"("append to file? (new file:F)"=TRUE, "1D data"=w515, "file path (dialog if empty)"=w514) -> ()  [unwired: 5 in, 1 out]
                  }
                }
                n187 = Multiply(x=0, y=w457) -> (x*y=w481:i32)
              }
            }
          }
        }
        n188 = Equal?(x=w158, y=0) -> (x = y?=w203:bool)
        n189 = case shown="True" w203 {
          tunnel: w176 -> [w293 w298]
          tunnel: w161 -> [_ _]
          tunnel: w160 -> [_ _]
          tunnel: w201 -> [_ w303]
          tunnel: w140 -> [w296 w302]
          tunnel: [w296 w301] -> w139
          tunnel: w181 -> [_ w300]
          tunnel: w180 -> [_ w299]
          tunnel: w118 -> [w292 _]
          tunnel: [w292 w297] -> w117
          frame False {
            n190 = property on="Property Node" class="XYGraph (strict)"(reference=w293, "Active Cursor"=u32 0, "Cursor.Visible"=FALSE) -> ()  [unwired: 1 in, 2 out]
          }
          frame True {
            n191 = case shown="True" w303 {
              tunnel: w302 -> [w311 w318]
              tunnel: [w311 w317] -> w301
              tunnel: w300 -> [w307 w322]
              tunnel: w299 -> [w306 w321]
              tunnel: w298 -> [_ _]
              tunnel: w298 -> [w305 w320]
              tunnel: [w304 w312] -> w297
              frame False {
                n192 = Bundle("x0"=w307, "y0"=w306) -> (w308:cluster{"x0":dbl, "y0":dbl})  [unwired: 1 in]
                n193 = invoke on="Invoke Node" class="XYGraph (strict)" method="Map XY To Coords"(reference=w305, "XY"=w308) -> ("Coords"=w304:T11)  [unwired: 5 in, 6 out]
                n194 = Unbundle(w304) -> ("Horizontal"=w310:i32, "Vertical"=w309:i32)
                n195 = dll-call lib="User32.dll" fn="SetCursorPos"(w310, w309) -> ()  [unwired: 6 in, 2 out]
              }
              frame True {
                n196 = Bundle("x0"=w322, "y0"=w321) -> (w314:cluster{"x0":dbl, "y0":dbl})  [unwired: 1 in]
                n197 = invoke on="Invoke Node" class="XYGraph (strict)" method="Map XY To Coords"(reference=w320, "XY"=w314) -> ("Coords"=w312:T11)  [unwired: 5 in, 6 out]
                n198 = Tick Count (ms)() -> (millisecond timer value=→"initial time":u32)
                n199 = Unbundle(w312) -> ("Horizontal"=w316:i32, "Vertical"=w315:i32)
                n200 = dll-call lib="User32.dll" fn="SetCursorPos"(w316, w315) -> ()  [unwired: 6 in, 2 out]
                n201 = Add(x=1, y=w318) -> (x+y=w317:i32)
              }
            }
          }
        }
        n202 = node-c288() -> ()  [unwired: 1 in, 1 out]
      }
      n203 = Open/Create/Replace File(file path (use dialog)=w90, operation (0:open)=T1."create") -> (refnum out=w92:refnum<file>)  [unwired: 4 in, 2 out]
      n204 = Open/Create/Replace File(file path (use dialog)=w84, operation (0:open)=T1."create") -> (refnum out=w86:refnum<file>)  [unwired: 4 in, 2 out]
      n205 = Open/Create/Replace File(file path (use dialog)=w73, operation (0:open)=T1."create") -> (refnum out=w74:refnum<file>)  [unwired: 4 in, 2 out]
      n206 = Open/Create/Replace File(file path (use dialog)=w70, operation (0:open)=T1."create") -> (refnum out=w71:refnum<file>)  [unwired: 4 in, 2 out]
      n207 = Open/Create/Replace File(file path (use dialog)=w87, operation (0:open)=T1."create") -> (refnum out=w89:refnum<file>)  [unwired: 4 in, 2 out]
      n208 = Close File(refnum=w92) -> ()  [unwired: 1 in, 2 out]
      n209 = Close File(refnum=w86) -> ()  [unwired: 1 in, 2 out]
      n210 = Close File(refnum=w74) -> ()  [unwired: 1 in, 2 out]
      n211 = Close File(refnum=w71) -> ()  [unwired: 1 in, 2 out]
      n212 = Close File(refnum=w89) -> ()  [unwired: 1 in, 2 out]
      n213 = node-c288(w98) -> ()  [unwired: 1 out]
      n214 = call-poly <vilib>:"Close Input Device.vi"("error in (no error)"=w81, "device ID"=w83) -> ()  [unwired: 8 in, 1 out]
    }
    frame #2 {
      n215 = call "finish.vi"("XYGraph Refnum"=w568) -> ()  [unwired: 11 in]
      n216 = call "Time Delay3"() -> ()  [unwired: 11 in, 1 out]
    }
  }
  n217 = property class="VI"(reference=w19, error in=w18, "Front Panel Window:Open"=TRUE) -> (reference out=w22:refnum<vi>, error out=w21:errorcluster)
  n218 = Close Reference(reference=w22, error in (no error)=w21) -> ()  [unwired: 1 out]
